vi "BuildSlaveRWr.vi"() -> (0 "RWr":i16[][](array[numeric]))   [LabVIEW 2018]
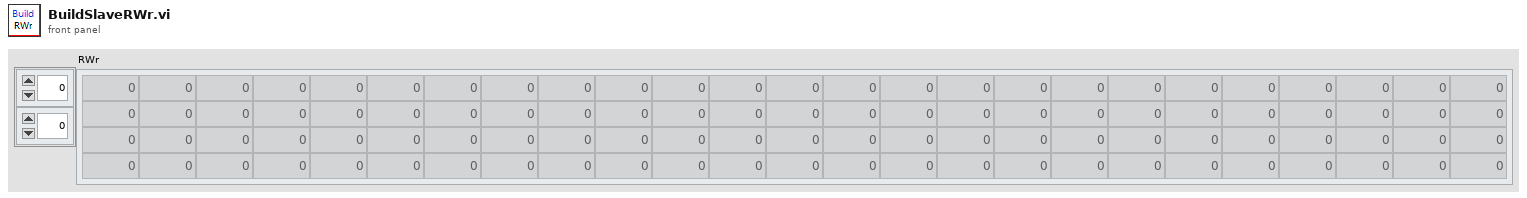
[diagram p1: front panel]
types:
  T1 = cluster{"轮盘预压力":sgl, "泄漏量上限":sgl, "压力上限":sgl, "压力下限":sgl, "风门闭电压上限":sgl, "风门闭电压下限":sgl, "风门开电压上限":sgl, "风门开电压下限":sgl, "LED电流上限":sgl, "LED电流下限":sgl, "气压稳定时间":sgl, "伺服速度":sgl, "INV初始频率":sgl, "INV变化周期":sgl, "INV慢速变化量":sgl, "INV快速变化量":sgl}
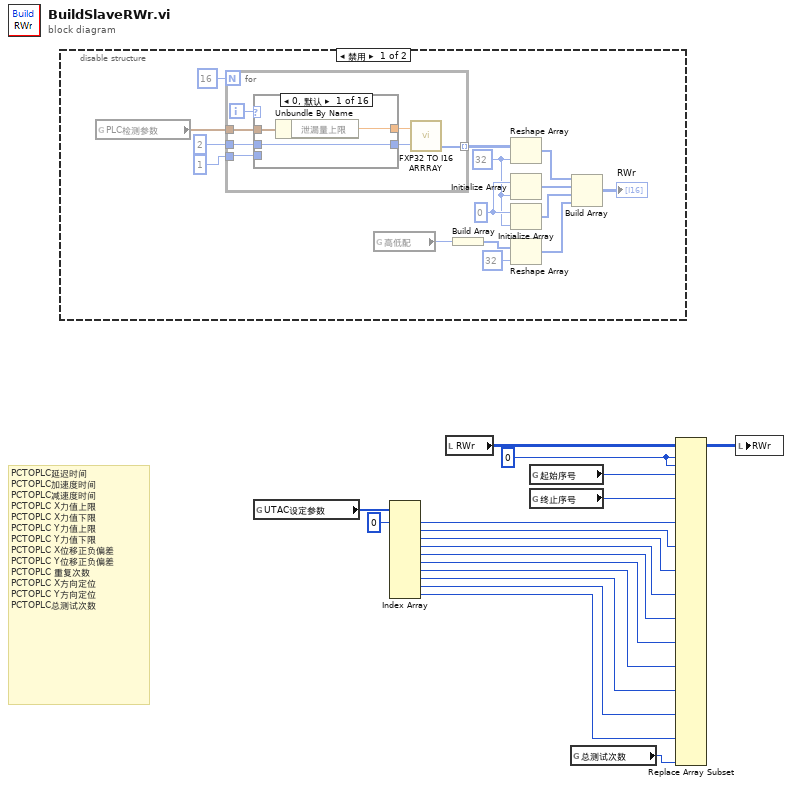
[diagram p0: block diagram]
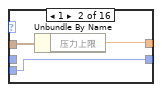
[diagram p2: hidden frame]
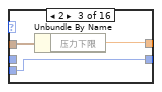
[diagram p3: hidden frame]
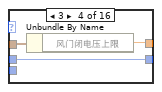
[diagram p4: hidden frame]
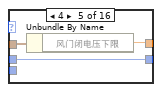
[diagram p5: hidden frame]
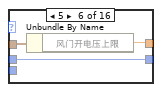
[diagram p6: hidden frame]
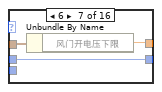
[diagram p7: hidden frame]
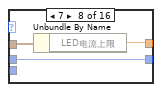
[diagram p8: hidden frame]
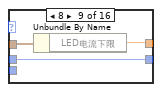
[diagram p9: hidden frame]
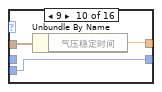
[diagram p10: hidden frame]
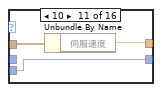
[diagram p11: hidden frame]
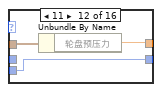
[diagram p12: hidden frame]
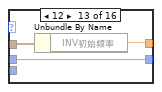
[diagram p13: hidden frame]
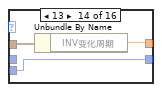
[diagram p14: hidden frame]
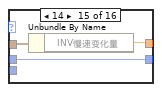
[diagram p15: hidden frame]
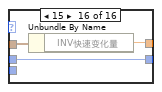
[diagram p16: hidden frame]
diagram:
  w2 = i16 0 ("索引 (行)")
  # "PCTOPLC延迟时间\nPCTOPLC加速度时间\nPCTOPLC减速度时间\nPCTOPLC X力值上限\nPCTOPLC X力值下限\nPCTOPLC Y力值上限\nPCTOPLC Y力值下限\nPCTOPLC X位移正负偏差\nPCTOPLC Y位移正负偏差\nPCTOPLC 重复次数\nPCTOPLC X方向定位\nPCTOPLC Y方向定位\nPCTOPLC总测试次数"
  n1 = disable-structure shown="禁用" {
    frame Disabled {
      w28 = i16 0
      w27 = 32 ("维数大小")
      n2 = global read "全局 1.vi" "PLC检测参数"() -> (w33:T1)
      n3 = for {
        N: 16 -> [_]
        tunnel: w33 -> [w40]
        tunnel: 2 ("位数(2)") -> [w39]
        tunnel: [w35] -> w29 mode=indexing
        tunnel: 1 ("位数(2)") -> [w34]
        i -> [w38]
        n4 = case shown="0, 默认" w38 {
          tunnel: w40 -> [w43 w46 w49 w52 w55 w58 w61 w64 w67 w70 w73 w76 w79 w82 w85 w88]
          tunnel: w39 -> [w41 _ _ w50 w53 w56 w59 w62 w65 _ _ _ w77 _ w83 w86]
          tunnel: [w42 w45 w48 w51 w54 w57 w60 w63 w66 w69 w72 w75 w78 w81 w84 w87] -> w37
          tunnel: [w41 w44 w47 w50 w53 w56 w59 w62 w65 w68 w71 w74 w77 w80 w83 w86] -> w36
          tunnel: w34 -> [_ w44 w47 _ _ _ _ _ _ w68 w71 w74 _ w80 _ _]
          frame 0, Default {
            n5 = Unbundle By Name(w43) -> ("泄漏量上限"=w42:sgl)
          }
          frame 1 {
            n6 = Unbundle By Name(w46) -> ("压力上限"=w45:sgl)
          }
          frame 2 {
            n7 = Unbundle By Name(w49) -> ("压力下限"=w48:sgl)
          }
          frame 3 {
            n8 = Unbundle By Name(w52) -> ("风门闭电压上限"=w51:sgl)
          }
          frame 4 {
            n9 = Unbundle By Name(w55) -> ("风门闭电压下限"=w54:sgl)
          }
          frame 5 {
            n10 = Unbundle By Name(w58) -> ("风门开电压上限"=w57:sgl)
          }
          frame 6 {
            n11 = Unbundle By Name(w61) -> ("风门开电压下限"=w60:sgl)
          }
          frame 7 {
            n12 = Unbundle By Name(w64) -> ("LED电流上限"=w63:sgl)
          }
          frame 8 {
            n13 = Unbundle By Name(w67) -> ("LED电流下限"=w66:sgl)
          }
          frame 9 {
            n14 = Unbundle By Name(w70) -> ("气压稳定时间"=w69:sgl)
          }
          frame 10 {
            n15 = Unbundle By Name(w73) -> ("伺服速度"=w72:sgl)
          }
          frame 11 {
            n16 = Unbundle By Name(w76) -> ("轮盘预压力"=w75:sgl)
          }
          frame 12 {
            n17 = Unbundle By Name(w79) -> ("INV初始频率"=w78:sgl)
          }
          frame 13 {
            n18 = Unbundle By Name(w82) -> ("INV变化周期"=w81:sgl)
          }
          frame 14 {
            n19 = Unbundle By Name(w85) -> ("INV慢速变化量"=w84:sgl)
          }
          frame 15 {
            n20 = Unbundle By Name(w88) -> ("INV快速变化量"=w87:sgl)
          }
        }
        n21 = call "FXP32 TO I16 ARRRAY.vi"("FXP32in"=w37, "位数(2)"=w36) -> ("out I16 array"=w35:i16[])  [unwired: 2 out]
      }
      n22 = global read "全局 1.vi" "高低配"() -> (w26:i16)
      n23 = Build Array(w26) -> (w25:i16[])
      n24 = Reshape Array ("重排数组维数")(w29, w27) -> (w21:i16[])
      n25 = Initialize Array(w28, w27) -> (w20:i16[])
      n26 = Initialize Array(w28, w27) -> (w19:i16[])
      n27 = Reshape Array(w25, 32 ("维数大小")) -> (w23:i16[])
      n28 = Build Array(w21, w20, w19, w23) -> (→"RWr":i16[][])
    }
    frame Enabled {
    }
  }
  n29 = global read "全局 1.vi" "UTAC设定参数"() -> (w18:i16[])
  n30 = Index Array(array=w18, index #1=i16 0 ("索引")) -> (element #1=w14:i16, element #2=w11:i16, element #3=w10:i16, element #4=w9:i16, element #5=w8:i16, element #6=w7:i16, element #7=w6:i16, element #8=w5:i16, element #9=w4:i16, element #10=w3:i16)  [unwired: 9 in]
  n31 = local read "RWr"() -> (w16:i16[][])
  n32 = global read "全局 1.vi" "起始序号"() -> (w13:i16)
  n33 = global read "全局 1.vi" "终止序号"() -> (w12:i16)
  n34 = global read "全局 1.vi" "总测试次数"() -> (w1:i16)
  n35 = Replace Array Subset(array=w16, new element #1=w13, index (row) #1=w2, index (col) #1=w2, new element #2=w12, new element #3=w14, new element #4=w11, new element #5=w10, new element #6=w9, new element #7=w8, new element #8=w7, new element #9=w6, new element #10=w5, new element #11=w4, new element #12=w3, new element #13=w1) -> (w15:i16[][])  [unwired: 24 in]
  n36 = local write "RWr"(w15) -> ()
